vi "File Path's.vi"(7 "Create New? (F)":bool, 11 "error in":errorcluster, 13 "File Name":T1) -> (8 "File Path Out":path, 15 "error out":errorcluster)   [LabVIEW 2024]
uses:
  Host-Control's/DTT File's Name.ctl
  8b54c3f3-cb5c-42ed-b762-c59440f849f3.vi
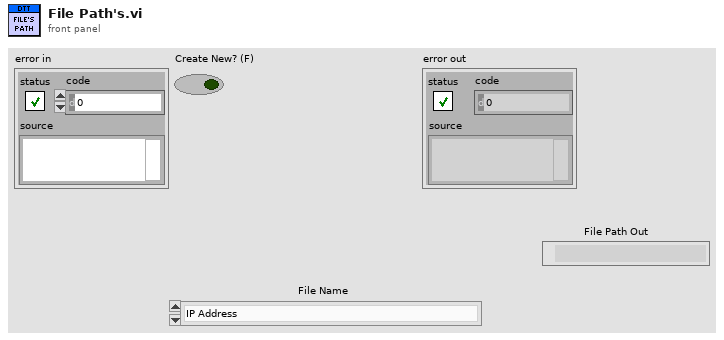
[diagram p1: front panel]
types:
  T1 = typedef "DTT File's Name.ctl" = enum16{"IP Address"}
  T2 = enum16{"open", "replace", "create", "open or create", "replace or create", "replace or create with confirmation"}
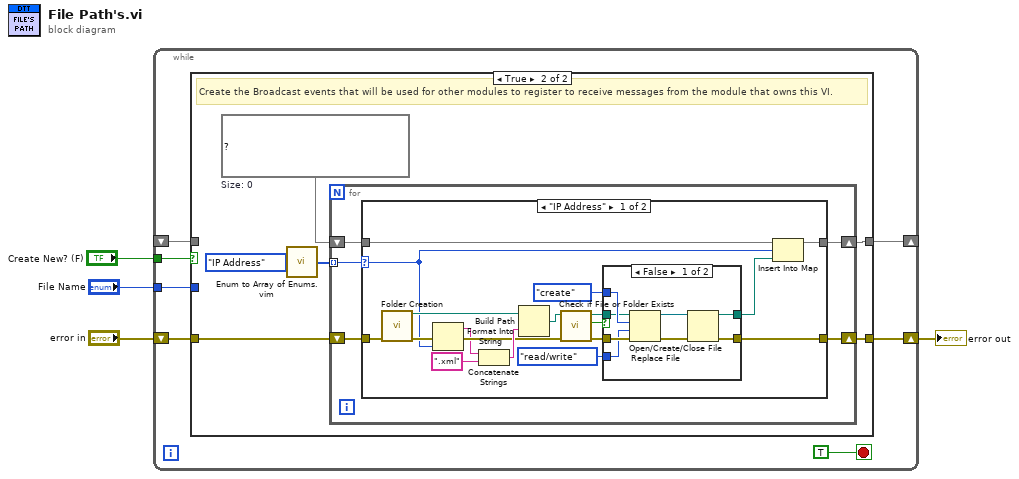
[diagram p0: block diagram]
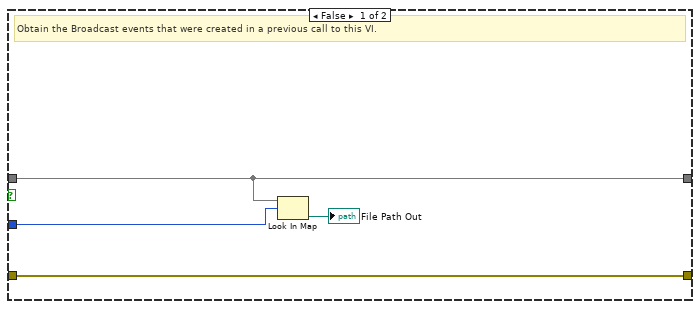
[diagram p2: hidden frame]
diagram:
  n1 = while {
    tunnel: "Create New? (F)" -> [w10]
    tunnel: "File Name" -> [w8]
    shift-right: [w9] -> w2
    shift-left: "error in" -> [w11]
    shift-right: [w7] -> _
    shift-left: _ -> [w6]
    stop <- TRUE stop-if-true
    n2 = case shown="True" w10 {
      tunnel: w11 -> [w13 w16]
      tunnel: [w15 w20] -> w7
      tunnel: w6 -> [w15 _]
      tunnel: [w13 w19] -> w9
      tunnel: w8 -> [w12 _]
      frame False {
        # "Obtain the Broadcast events that were created in a previous call to this VI."
        n3 = Look In Map(map=w15, key=w12) -> (value=→"File Path Out":path)  [unwired: 1 in, 1 out]
      }
      frame True {
        w21 = map{T1, path} {}  # Size: 0
        # "Create the Broadcast events that will be used for other modules to register to receive messages from the module that owns this VI."
        n4 = call "Enum to Array of Enums.vim"("enum"=DTT_File's_Name."IP Address" ("File Name")) -> ("array of enums"=w18:T1[])
        n5 = for {
          shift-right: [w26] -> w19
          shift-left: w16 -> [w23]
          shift-right: [w24] -> w20
          shift-left: w21 -> [w25]
          tunnel: w18 -> [w22] mode=indexing
          n6 = case shown="\"IP Address\"" w22 {
            selector: w22 -> [w37 _]
            tunnel: [w27 w55] -> w26
            tunnel: w25 -> [w44 w56]
            tunnel: [w43 w56] -> w24
            tunnel: w23 -> [w42 w55]
            frame "IP Address" {
              n7 = call "Folder Creation.vi"("error in"=w42) -> ("Tower Test File's - Folder Path"=w40:path, "error out"=w41:errorcluster)  [unwired: 12 in, 1 out]
              n8 = Format Into String(error in=w41, w37) -> (resulting string=w32:string, error out=w35:errorcluster)  [unwired: 2 in]
              n9 = Concatenate Strings(w32, ".xml" ("string")) -> (w38:string)
              n10 = Build Path(base path=w40, name or relative path=w38) -> (appended path=w36:path)
              n11 = call <vilib>:"Check if File or Folder Exists.vi"("error in (no error)"=w35, "path"=w36) -> ("error out"=w33:errorcluster, "file or folder exists?"=w34:bool, "dup path"=w31:path)  [unwired: 7 in]
              n12 = case shown="False" w34 {
                tunnel: w33 -> [w50 w53]
                tunnel: w31 -> [w51 w54]
                tunnel: [w45 w54] -> w30
                tunnel: T2."create" ("operation (0:open)") -> [w52 _]
                tunnel: enum16{"read/write", "read-only", "write-only"}."read/write" ("access (0:read/write)") -> [w49 _]
                tunnel: [w46 w53] -> w27
                frame False {
                  n13 = Open/Create/Replace File(file path (use dialog)=w51, error in=w50, operation (0:open)=w52, access (0:read/write)=w49) -> (refnum out=w48:refnum<file>, error out=w47:errorcluster)  [unwired: 2 in, 1 out]
                  n14 = Close File(refnum=w48, error in=w47) -> (path=w45:path, error out=w46:errorcluster)
                }
                frame True {
                }
              }
              n15 = Insert Into Map(map in=w44, key=w37, value=w30) -> (map out=w43:map{T1, path})  [unwired: 2 out]
            }
            frame Default {
            }
          }
        }
      }
    }
  }
  "error out" <- w2
